vi "找出数组中元素的位置.vi"(10 "元素":string, 11 "数组":string[](array[string])) -> (3 "数组 2":i32[](array[numeric]))   [LabVIEW 2017]
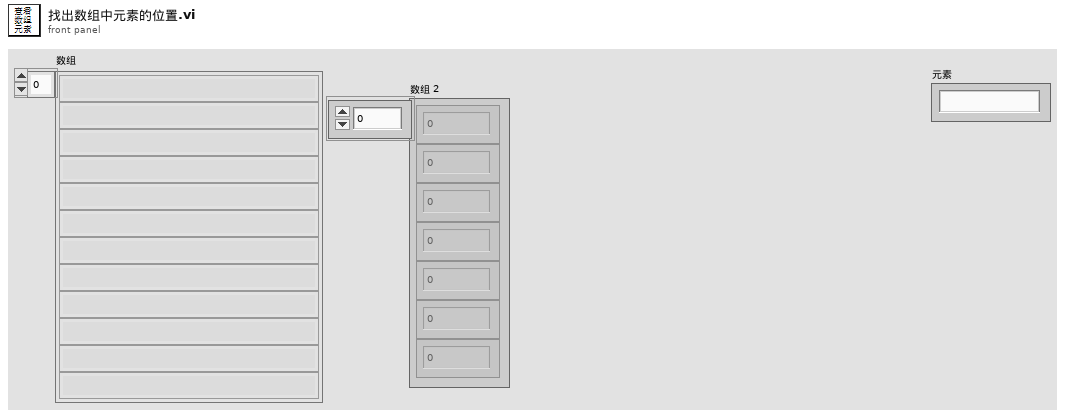
[diagram p1: front panel]
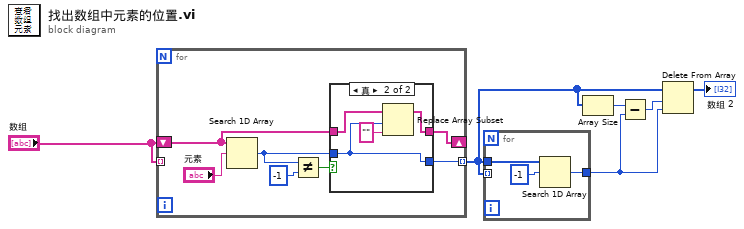
[diagram p0: block diagram]
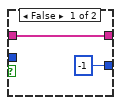
[diagram p2: hidden frame]
diagram:
  n1 = for {
    tunnel: "数组" -> [_] mode=indexing
    tunnel: [w10] -> w5 mode=indexing
    shift-right: [w7] -> _
    shift-left: "数组" -> [w9]
    n2 = Search 1D Array(1D array=w9, element="元素") -> (index of element=w8:i32)  [unwired: 1 in]
    n3 = Not Equal?(x=w8, y=-1) -> (x != y?=w11:bool)
    n4 = case shown="真" w11 {
      tunnel: [-1 w17] -> w10
      tunnel: w9 -> [w14 w19]
      tunnel: w8 -> [_ w17]
      tunnel: [w14 w18] -> w7
      frame False {
      }
      frame True {
        n5 = Replace Array Subset(array=w19, new element="" ("新元素/子数组"), index=w17) -> (w18:string[])
      }
    }
  }
  n6 = for {
    tunnel: w5 -> [_] mode=indexing
    tunnel: w5 -> [w22]
    tunnel: [w20] -> w4
    n7 = Search 1D Array(1D array=w22, element=-1 ("元素")) -> (index of element=w20:i32)  [unwired: 1 in]
  }
  n8 = Array Size(array=w5) -> (size(s)=w2:i32)
  n9 = Subtract(x=w2, y=w4) -> (x-y=w3:i32)
  n10 = Delete From Array(array=w5, length=w3, index=w4) -> (array with subset deleted=→"数组 2":i32[])  [unwired: 1 out]
